vi "Main.vi"() -> ()   [LabVIEW 2013]
doc: "This template is for the Queued Message Handler design pattern.\n\nThe Event Handling Loop generates messages based on user interface actions.\n\nThe Message Handling Loop processes messages generated by the Event Handling Loop, or by other messages. The messages are string values, so new messages can be added easily to the Message Cases case structure in the Message Handling Loop. Each message cluster can also provide an optional value for Message Data, which is a variant that can be converted to whatever message-specific data is required."
uses:
  <instrlib>/niHSDIO/niHSDIO.llb/niHSDIO_ctl Voltage Logic Family Values (Ring).ctl
  Controls/USID.ctl
  Controls/Reg_Address_Data.ctl
  Manual Control/controls/UI Data.ctl
  Manual Control/support/Message Queue/Enqueue Message (Single).vi
  Manual Control/support/Message Queue/Enqueue Message (Array).vi
  <vilib>/Utility/error.llb/Error Cluster From Error Code.vi
  <vilib>/ErrorRing/Error Ring.xnode
  Manual Control/support/Message Queue/Message Queue.lvlib
  Manual Control/support/User Event - Stop/User Event - Stop.lvlib
panel:
  in  "Tab Control":enum32{"Setup", "Run"}(tab)
  in  "Initialize Instrument":bool
  in  "HDSIO_PPMU_Settings":T1={"voltage level"=1.8, "current range"=0.002, "aperture time (4E-6 s)"=0.01667} {"aperture time (4E-6 s)" format="%#_6p"; "current range" format="%#_6p"}
  in  "HDSIO_Settings":T3={"HSDIO VISA"="6556_0", "logic family "=8, "Clock Rate"=40000000.0, "channel list (Clock,Data)"="0"} {"Clock Rate" format="%.2p"; "logic family" items=["5.0V Logic"=5, "3.3V Logic"=6, "2.5V Logic"=7, "1.8V Logic"=8, "1.5V Logic"=80, "1.2V Logic"=81]}
  in  "OVS":u8=16
  in  "sample rate":dbl=20000000.0 format="%#_13p"
  in  "Write SuBUS":bool
  in  "Measure Current":bool
  out "voltage measurements":dbl[](array[numeric]) format="%#_6p"
  out "current measurements":dbl[](array[numeric]) format="%#_6p"
  in  "USID":T4=13 max=15
  in  "Reg_Address_Data":T5={"Address"=81, "Data"=0} {"Address" format="%.0x"}
  out "Display <Replace Me>":string
  in  "Exit":bool
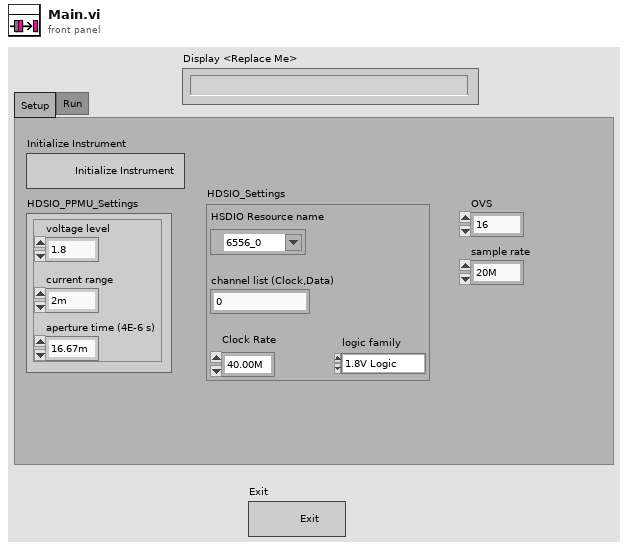
[diagram p1: front panel]
types:
  T1 = cluster{"voltage level":dbl, "current range":dbl, "aperture time (4E-6 s)":dbl}
  T2 = typedef "niHSDIO_ctl Voltage Logic Family Values (Ring).ctl" = i32
  T3 = cluster{"HSDIO VISA":refnum<k15>, "logic family ":T2, "Clock Rate":dbl, "channel list (Clock,Data)":string}
  T4 = typedef "USID.ctl" = u8
  T5 = typedef "Reg_Address_Data.ctl" = cluster{"Address":u8, "Data":u8}
  T6 = cluster{"HSDIO_ACQ":refnum<k15>, "HSDIO_GEN":refnum<k15>}
  T7 = typedef "UI Data.ctl" = cluster{"Boolean <Replace Me>":bool, "String <Replace Me>":string, "Numeric <Replace Me>":dbl, "Do Something Ref":refnum<vi>, "Do Something Else Ref":refnum<vi>, "Data Display Ref":refnum<vi>, "Exit Button Ref":refnum<vi>}
  T8 = typedef "Message Queue.lvlib/All Message Queues.ctl" = cluster{"UI":refnum<queue>}
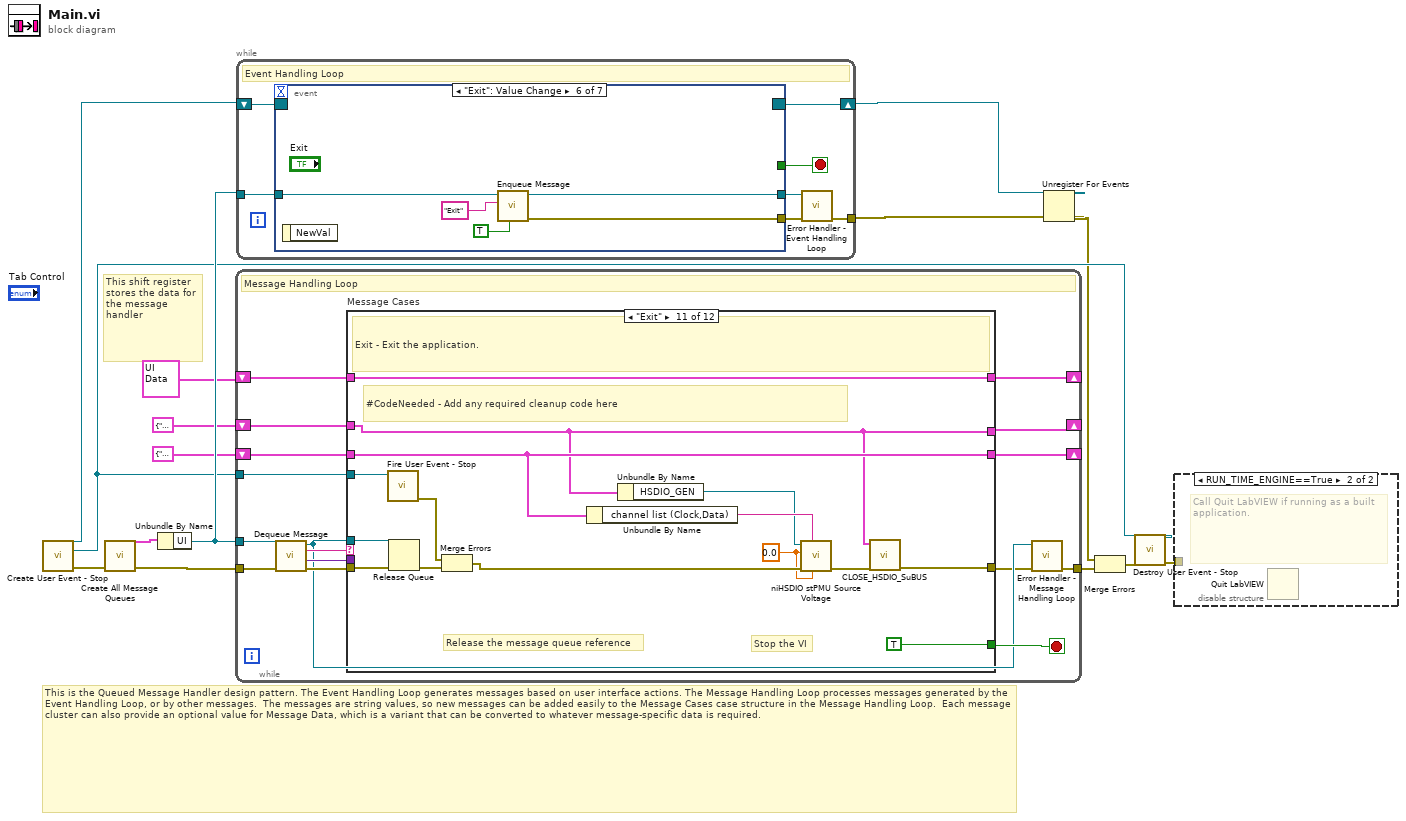
[diagram p0: block diagram]
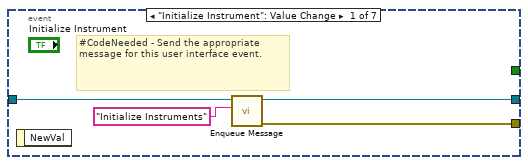
[diagram p3: hidden frame]
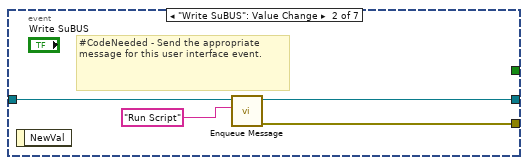
[diagram p4: hidden frame]
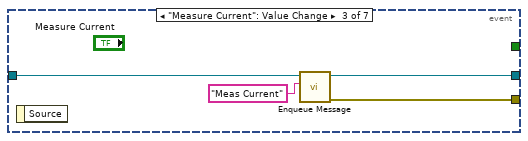
[diagram p5: hidden frame]
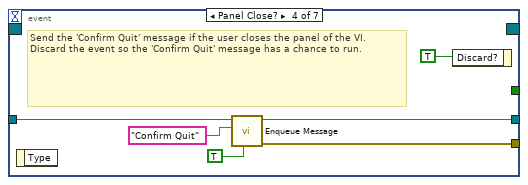
[diagram p6: hidden frame]
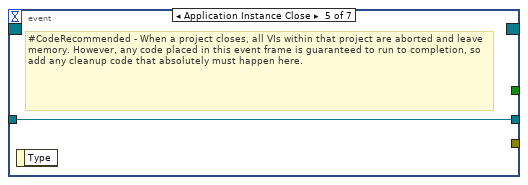
[diagram p7: hidden frame]
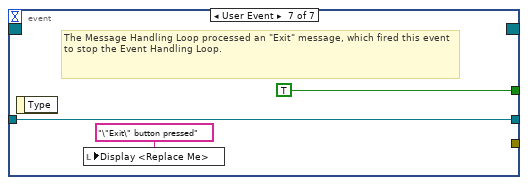
[diagram p8: hidden frame]
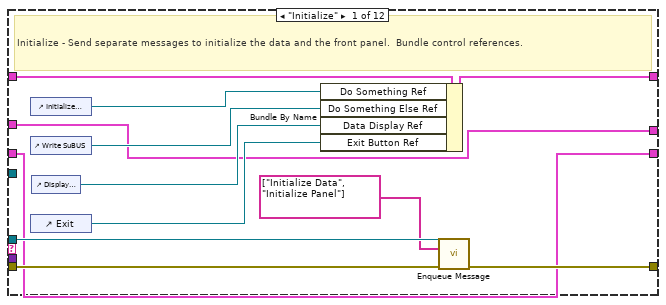
[diagram p9: hidden frame]
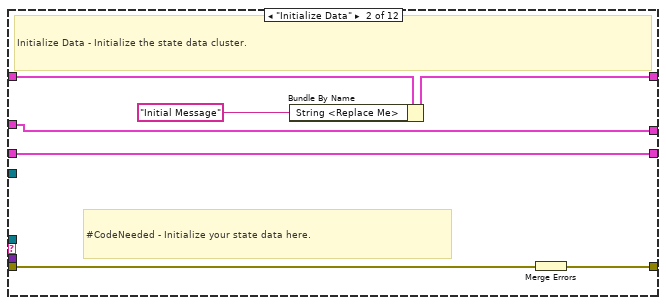
[diagram p10: hidden frame]
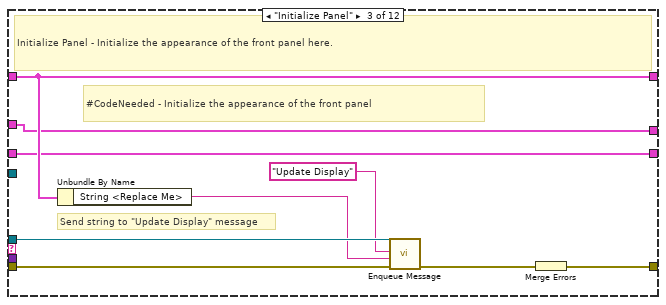
[diagram p11: hidden frame]
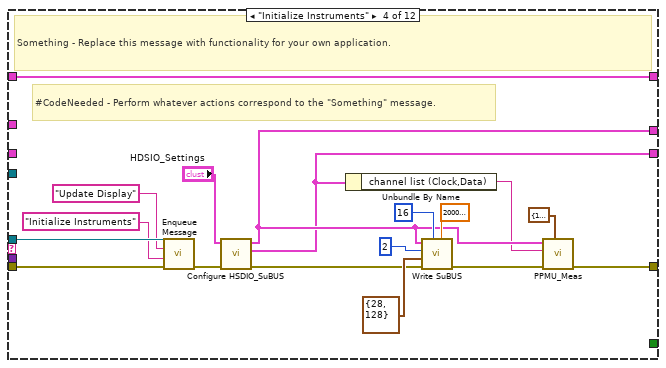
[diagram p12: hidden frame]
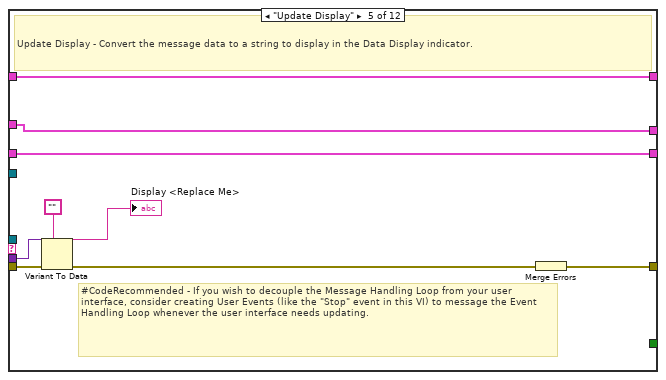
[diagram p13: hidden frame]
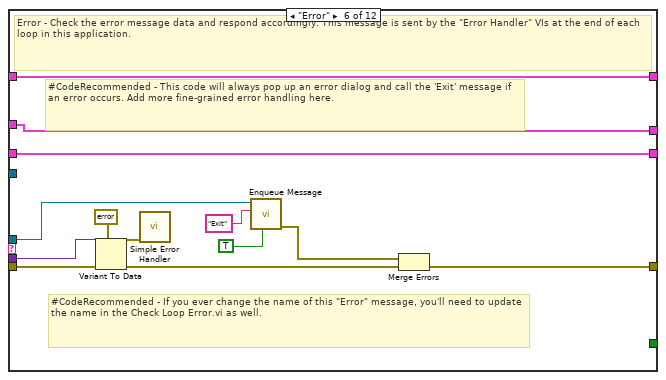
[diagram p14: hidden frame]
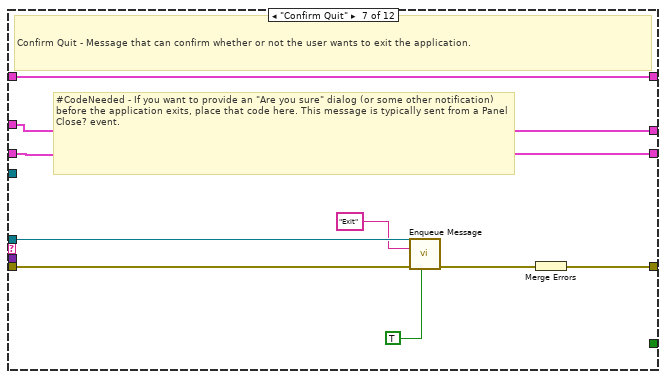
[diagram p15: hidden frame]
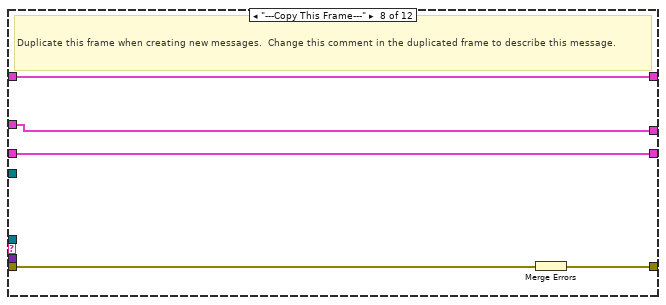
[diagram p16: hidden frame]
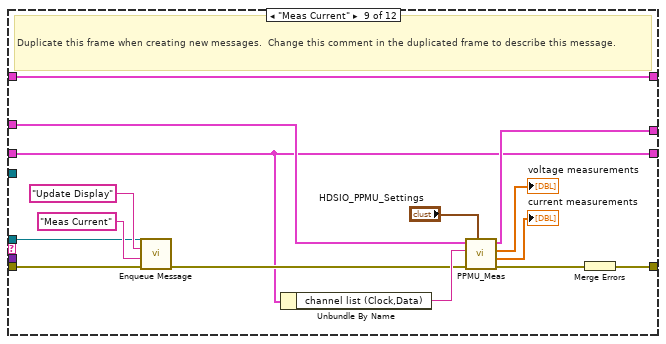
[diagram p17: hidden frame]
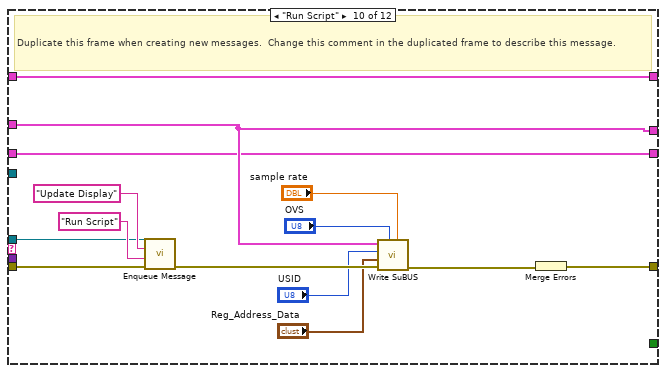
[diagram p18: hidden frame]
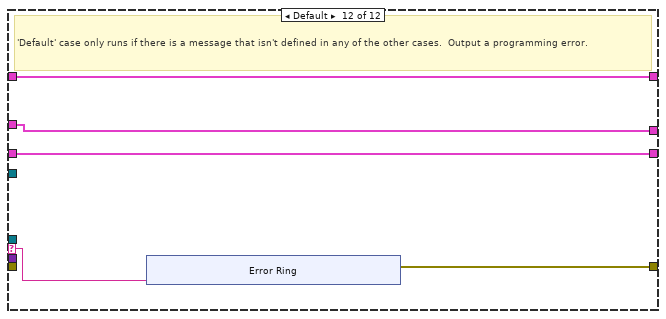
[diagram p19: hidden frame]
diagram:
  # "This is the Queued Message Handler design pattern. The Event Handling Loop generates messages based on user interface actions. The Message Handling Loop processes messages generated by the Event Handling Loop, or by other messages.  The messages are string values, so new messages can be added easily to the Message Cases case structure in the Message Handling Loop.  Each message cluster can also provide an optional value for Message Data, which is a variant that can be converted to whatever message-specific data is required."
  # "This shift register stores the data for the message handler"
  n1 = call "Create User Event - Stop.vi"() -> ("error out"=w10:errorcluster, "User Event - Stop"=w8:refnum<user-event>, "Stop Event Registration Refnum"=w11:refnum<event-registration>)  [unwired: 9 in]
  n2 = call "Create All Message Queues.vi"("error in (no error)"=w10) -> ("error out"=w15:errorcluster, "Message Queues out"=w14:T8)  [unwired: 9 in]
  n3 = Unbundle By Name(w14) -> ("UI"=w12:refnum<queue>)
  n4 = while {
    tunnel: w12 -> [w23]
    shift-right: [w30] -> _
    shift-left: T7 {"Boolean <Replace Me>"=FALSE, "String <Replace Me>"="", "Numeric <Replace Me>"=0.0, "Do Something Ref"=refnum, "Do Something Else Ref"=refnum, "Data Display Ref"=refnum, "Exit Button Ref"=refnum} ("Data Cluster") -> [w31]
    tunnel: w8 -> [w28]
    tunnel: w15 -> [w27]
    tunnel: [w21] -> w13
    shift-right: [w19] -> _
    shift-left: T3 {"HSDIO VISA"="", "logic family "=0, "Clock Rate"=0.0, "channel list (Clock,Data)"=""} ("HDSIO_Settings 2") -> [w18]
    shift-right: [w17] -> _
    shift-left: T6 {"HSDIO_ACQ"="", "HSDIO_GEN"=""} ("HSDIO Sessions") -> [w16]
    stop <- w29 stop-if-true
    # "Message Handling Loop"
    n5 = call "Dequeue Message.vi"("error in (no error)"=w27, "Message Queue"=w23) -> ("error out"=w26:errorcluster, "Message Data"=w24:variant, "Message"=w25:string, "dup Message Queue"=w22:refnum<queue>)  [unwired: 6 in]
    n6 = case "Message Cases" shown="\"Exit\"" w25 {
      selector: w25 -> [_ _ _ _ _ _ _ _ _ _ _ w160]
      tunnel: w22 -> [w41 _ w56 w75 _ w91 w104 _ w123 w137 w157 _]
      tunnel: w26 -> [w42 w50 w57 w76 w84 w99 w108 w113 w124 w139 w153 _]
      tunnel: [w43 w46 w58 w69 w85 w92 w106 w111 w127 w141 w150 w161] -> w20
      tunnel: w31 -> [w40 w49 w59 w77 w86 w98 w107 w112 w128 w142 w156 w162]
      tunnel: [w39 w48 w59 w77 w86 w98 w107 w112 w128 w142 w156 w162] -> w30
      tunnel: [_ _ _ _ _ _ _ _ _ _ TRUE _] -> w29
      tunnel: w24 -> [_ _ _ _ w83 w97 _ _ _ _ _ _]
      tunnel: w28 -> [_ _ _ _ _ _ _ _ _ _ w152 _]
      tunnel: [w33 w45 w52 w61 w79 w88 w101 w110 w114 w129 w149 w159] -> w19
      tunnel: w18 -> [w33 w45 w52 _ w79 w88 w101 w110 w114 w129 w149 w159]
      tunnel: [w32 w44 w51 w62 w78 w87 w100 w109 w115 w130 w148 w158] -> w17
      tunnel: w16 -> [w32 w44 w51 _ w78 w87 w100 w109 w116 w130 w148 w158]
      frame "Initialize" {
        # "Initialize - Send separate messages to initialize the data and the front panel.  Bundle control references."
        n7 = control-ref of="Initialize Instrument"() -> (w38:refnum<vi>)
        n8 = control-ref of="Write SuBUS"() -> (w37:refnum<vi>)
        n9 = control-ref of="Exit"() -> (w35:refnum<vi>)
        n10 = control-ref of="Display <Replace Me>"() -> (w36:refnum<vi>)
        n11 = Bundle By Name(cluster=w40, "Do Something Ref"=w38, "Do Something Else Ref"=w37, "Data Display Ref"=w36, "Exit Button Ref"=w35) -> (w39:T7)
        n12 = call-poly "Enqueue Message.vi"("error in (no error)"=w42, "Message Array"=string[] ["Initialize Data", "Initialize Panel"], "Message Queue"=w41) -> ("error out"=w43:errorcluster)  [unwired: 7 in, 1 out]
      }
      frame "Initialize Data" {
        # "#CodeNeeded - Initialize your state data here."
        # "Initialize Data - Initialize the state data cluster."
        n13 = Bundle By Name(cluster=w49, "String <Replace Me>"="Initial Message" ("Initial Message")) -> (w48:T7)
        n14 = Merge Errors(w50) -> (w46:errorcluster)
      }
      frame "Initialize Panel" {
        # "Send string to \"Update Display\" message"
        # "#CodeNeeded - Initialize the appearance of the front panel"
        # "Initialize Panel - Initialize the appearance of the front panel here."
        n15 = Unbundle By Name(w59) -> ("String <Replace Me>"=w53:string)
        n16 = call-poly "Enqueue Message.vi"("error in (no error)"=w57, "Message Data"=w53, "Message"="Update Display", "Message Queue"=w56) -> ("error out"=w55:errorcluster)  [unwired: 6 in, 1 out]
        n17 = Merge Errors(w55) -> (w58:errorcluster)
      }
      frame "Initialize Instruments" {
        # "#CodeNeeded - Perform whatever actions correspond to the \"Something\" message."
        # "Something - Replace this message with functionality for your own application."
        n18 = call-poly "Enqueue Message.vi"("error in (no error)"=w76, "Message Data"="Initialize Instruments" ("\"Do Something\" button pressed"), "Message"="Update Display", "Message Queue"=w75) -> ("error out"=w72:errorcluster)  [unwired: 6 in, 1 out]
        n19 = call "Configure HSDIO_SuBUS.vi"("error in (no error)"=w72, "HDSIO_Settings"="HDSIO_Settings") -> ("error out"=w63:errorcluster, "HDSIO_Settings 2"=w61:T3, "HSDIO Sessions"=w62:T6)  [unwired: 7 in]
        n20 = Unbundle By Name(w61) -> ("channel list (Clock,Data)"=w60:string)
        n21 = call "Write SuBUS.vi"("sample rate"=20000000.0, "OVS"=u8 16, "Error In"=w63, "Reg_Address_Data"=T5 {"Address"=28, "Data"=128}, "USID"=T4 2, "HSDIO Sessions"=w62) -> ("Error Out"=w64:errorcluster)  [unwired: 5 in]
        n22 = call "PPMU_Meas.vi"("HDSIO_PPMU_Settings"=T1 {"voltage level"=1.8, "current range"=0.0, "aperture time (4E-6 s)"=4e-06}, "Error In"=w64, "channel list"=w60, "HSDIO Sessions"=w62) -> ("Error Out"=w69:errorcluster)  [unwired: 4 in, 3 out]
      }
      frame "Update Display" {
        # "#CodeRecommended - If you wish to decouple the Message Handling Loop from your user interface, consider creating User Events (like the \"Stop\" event in this VI) to message the Event Handling Loop whenever the user interface needs updating."
        # "Update Display - Convert the message data to a string to display in the Data Display indicator."
        n23 = Variant To Data(error in=w84, type="", Variant=w83) -> (data=→"Display <Replace Me>":string, error out=w81:errorcluster)
        n24 = Merge Errors(w81) -> (w85:errorcluster)
      }
      frame "Error" {
        # "#CodeRecommended - If you ever change the name of this \"Error\" message, you'll need to update the name in the Check Loop Error.vi as well."
        # "#CodeRecommended - This code will always pop up an error dialog and call the 'Exit' message if an error occurs. Add more fine-grained error handling here."
        # "Error - Check the error message data and respond accordingly. This message is sent by the \"Error Handler\" VIs at the end of each loop in this application."
        n25 = Variant To Data(error in=w99, type=errorcluster {"status"=FALSE, "code"=0, "source"=""} ("error constant"), Variant=w97) -> (data=w95:errorcluster, error out=w94:errorcluster)
        n26 = call <vilib>:"Simple Error Handler.vi"("error in (no error)"=w95) -> ()  [unwired: 4 in, 5 out]
        n27 = call-poly "Enqueue Message.vi"("Priority Message? (F)"=TRUE, "Message"="Exit", "Message Queue"=w91) -> ("error out"=w93:errorcluster)  [unwired: 7 in, 1 out]
        n28 = Merge Errors(w93, w94) -> (w92:errorcluster)
      }
      frame "Confirm Quit" {
        # "#CodeNeeded - If you want to provide an \"Are you sure\" dialog (or some other notification) before the application exits, place that code here. This message is typically sent from a Panel Close? event."
        # "Confirm Quit - Message that can confirm whether or not the user wants to exit the application."
        n29 = call-poly "Enqueue Message.vi"("Priority Message? (F)"=TRUE, "error in (no error)"=w108, "Message"="Exit", "Message Queue"=w104) -> ("error out"=w105:errorcluster)  [unwired: 6 in, 1 out]
        n30 = Merge Errors(w105) -> (w106:errorcluster)
      }
      frame "---Copy This Frame---" {
        # "Duplicate this frame when creating new messages.  Change this comment in the duplicated frame to describe this message."
        n31 = Merge Errors(w113) -> (w111:errorcluster)
      }
      frame "Meas Current" {
        # "Duplicate this frame when creating new messages.  Change this comment in the duplicated frame to describe this message."
        n32 = call-poly "Enqueue Message.vi"("error in (no error)"=w124, "Message Data"="Meas Current" ("\"Do Something\" button pressed"), "Message"="Update Display", "Message Queue"=w123) -> ("error out"=w117:errorcluster)  [unwired: 6 in, 1 out]
        n33 = Unbundle By Name(w114) -> ("channel list (Clock,Data)"=w121:string)
        n34 = call "PPMU_Meas.vi"("HDSIO_PPMU_Settings"="HDSIO_PPMU_Settings", "Error In"=w117, "channel list"=w121, "HSDIO Sessions"=w116) -> ("Error Out"=w122:errorcluster, "current measurements"=→"current measurements":dbl[], "voltage measurements"=→"voltage measurements":dbl[], "HSDIO Sessions"=w115:T6)  [unwired: 4 in]
        n35 = Merge Errors(w122) -> (w127:errorcluster)
      }
      frame "Run Script" {
        # "Duplicate this frame when creating new messages.  Change this comment in the duplicated frame to describe this message."
        n36 = call-poly "Enqueue Message.vi"("error in (no error)"=w139, "Message Data"="Run Script" ("\"Do Something\" button pressed"), "Message"="Update Display", "Message Queue"=w137) -> ("error out"=w135:errorcluster)  [unwired: 6 in, 1 out]
        n37 = call "Write SuBUS.vi"("sample rate"="sample rate", "OVS"="OVS", "Error In"=w135, "Reg_Address_Data"="Reg_Address_Data", "USID"="USID", "HSDIO Sessions"=w130) -> ("Error Out"=w136:errorcluster)  [unwired: 5 in]
        n38 = Merge Errors(w136) -> (w141:errorcluster)
      }
      frame "Exit" {
        w143 = 0.0 ("high level (3.30 volts)")
        # "Stop the VI"
        # "Release the message queue reference"
        # "#CodeNeeded - Add any required cleanup code here"
        # "Exit - Exit the application."
        n39 = call "Fire User Event - Stop.vi"("User Event - Stop"=w152) -> ("error out"=w151:errorcluster)  [unwired: 10 in]
        n40 = Release Queue(queue=w157, error in (no error)=w153) -> (error out=w154:errorcluster)  [unwired: 1 in, 2 out]
        n41 = Merge Errors(w151, w154) -> (w146:errorcluster)
        n42 = Unbundle By Name(w149) -> ("channel list (Clock,Data)"=w145:string)
        n43 = Unbundle By Name(w148) -> ("HSDIO_GEN"=w144:refnum<k15>)
        n44 = call <instrlib>:"niHSDIO stPMU Source Voltage.vi"("current range"=w143, "channel list"=w145, "error in (no error)"=w146, "voltage level"=w143, "instrument handle"=w144) -> ("error out"=w147:errorcluster)  [unwired: 5 in, 1 out]
        n45 = call "CLOSE_HSDIO_SuBUS.vi"("Error In"=w147, "HSDIO Sessions"=w148) -> ("Error Out"=w150:errorcluster)  [unwired: 9 in]
      }
      frame Default {
        # "'Default' case only runs if there is a message that isn't defined in any of the other cases.  Output a programming error."
        n46 = xnode "Error Ring"("parameter 0"=w160) -> ("error out"=w161:errorcluster)
      }
    }
    n47 = call "Error Handler - Message Handling Loop.vi"("error in (no error)"=w20, "Message Queue"=w22) -> ("dup error in"=w21:errorcluster)  [unwired: 8 in, 1 out]
  }
  n48 = while {
    tunnel: w12 -> [w176]
    shift-right: [w174] -> w6
    shift-left: w11 -> [w175]
    tunnel: [w170] -> w3
    stop <- w172 stop-if-true
    # "Event Handling Loop"
    n49 = event shown="[5] \"Exit\": Value Change" {
      selector: w175 -> [_ _ _ _ _ _ _]
      dyn-events: [_ _ _ _ _ _ _] -> w174
      timeout: _ -> [_ _ _ _ _ _ _]
      tunnel: [_ _ _ _ _ _ TRUE ("Discard?")] -> w172
      tunnel: w176 -> [w180 w184 w187 w193 w195 w200 w203]
      tunnel: [w177 w181 w185 w192 _ w199 _] -> w173
      tunnel: [w179 w183 w186 w191 w195 w198 w203] -> w171
      event "Initialize Instrument": Value Change {
        # "#CodeNeeded - Send the appropriate message for this user interface event."
        n50 = event-data() -> ()  [unwired: 1 in, 1 out]
        n51 = call-poly "Enqueue Message.vi"("Message"="Initialize Instruments", "Message Queue"=w180) -> ("error out"=w177:errorcluster, "dup Message Queue"=w179:refnum<queue>)  [unwired: 8 in]
      }
      event "Write SuBUS": Value Change {
        # "#CodeNeeded - Send the appropriate message for this user interface event."
        n52 = event-data() -> ()  [unwired: 1 in, 1 out]
        n53 = call-poly "Enqueue Message.vi"("Message"="Run Script", "Message Queue"=w184) -> ("error out"=w181:errorcluster, "dup Message Queue"=w183:refnum<queue>)  [unwired: 8 in]
      }
      event "Measure Current": Value Change {
        n54 = event-data() -> ()  [unwired: 1 in, 1 out]
        n55 = call-poly "Enqueue Message.vi"("Message"="Meas Current", "Message Queue"=w187) -> ("error out"=w185:errorcluster, "dup Message Queue"=w186:refnum<queue>)  [unwired: 8 in]
      }
      event Panel Close? {
        # "Send the 'Confirm Quit' message if the user closes the panel of the VI. Discard the event so the 'Confirm Quit' message has a chance to run."
        n56 = event-data() -> ()  [unwired: 1 in, 1 out]
        n57 = call-poly "Enqueue Message.vi"("Priority Message? (F)"=TRUE, "Message"="Confirm Quit", "Message Queue"=w193) -> ("error out"=w192:errorcluster, "dup Message Queue"=w191:refnum<queue>)  [unwired: 7 in]
        n58 = event-data("Discard?"=TRUE) -> ()  [unwired: 1 in, 1 out]
      }
      event Application Instance Close {
        # "#CodeRecommended - When a project closes, all VIs within that project are aborted and leave memory. However, any code placed in this event frame is guaranteed to run to completion, so add any cleanup code that absolutely must happen here."
        n59 = event-data() -> ()  [unwired: 1 in, 1 out]
      }
      event "Exit": Value Change {
        n60 = event-data() -> ()  [unwired: 1 in, 1 out]
        n61 = call-poly "Enqueue Message.vi"("Priority Message? (F)"=TRUE, "Message"="Exit", "Message Queue"=w200) -> ("error out"=w199:errorcluster, "dup Message Queue"=w198:refnum<queue>)  [unwired: 7 in]
      }
      event User Event {
        # "The Message Handling Loop processed an \"Exit\" message, which fired this event to stop the Event Handling Loop."
        n62 = event-data() -> ()  [unwired: 1 in, 1 out]
        n63 = local write "Display <Replace Me>"("\"Exit\" button pressed" ("VI Stopped")) -> ()
      }
    }
    n64 = call "Error Handler - Event Handling Loop.vi"("error in (no error)"=w173, "Message Queue"=w171) -> ("dup error in"=w170:errorcluster)  [unwired: 8 in, 1 out]
  }
  n65 = Unregister For Events(event registration refnum=w6, error in=w3) -> (error out=w7:errorcluster)
  n66 = Merge Errors(w7, w13) -> (w9:errorcluster)
  n67 = call "Destroy User Event - Stop.vi"("error in (no error)"=w9, "User Event - Stop"=w8) -> ("error out"=w4:errorcluster)  [unwired: 9 in]
  n68 = disable-structure shown="RUN_TIME_ENGINE==True" {
    disable-tunnel: w4 -> [_ _]
    frame condition #0 (active) {
    }
    frame condition #1 {
      # "Call Quit LabVIEW if running as a built application."
      n69 = Quit LabVIEW() -> ()  [unwired: 1 in]
    }
  }
